vi "Intake Loop.vi"(8 "error in (no error)":errorcluster) -> ()   [LabVIEW 2014]
uses:
  Intake Control.ctl
  <vilib>/Rock Robotics/WPI/MotorControl/WPI_MotorControlDeviceRef.ctl
  <vilib>/Rock Robotics/SystemInterfaces/Typedef/FPGA_TypedefDigitalModule.ctl
  <vilib>/Rock Robotics/SystemInterfaces/DIO/FPGA_DIOPWMChannel.ctl
  <vilib>/Rock Robotics/WPI/PWM/WPI_PWMDeadband.ctl
  <vilib>/Rock Robotics/WPI/CAN/Jaguar/SubVIs/WPI_CANJaguar_ControlMode.ctl
  <vilib>/Rock Robotics/WPI/PWM/WPI_PWMTransform_ConPane.ctl
  <vilib>/Rock Robotics/WPI/Solenoid/WPI_SolenoidDevRef.ctl
  <vilib>/Rock Robotics/SystemInterfaces/Typedef/FPGA_TypedefSolenoidModule.ctl
  <vilib>/Rock Robotics/WPI/Solenoid/WPI_SolenoidChannel.ctl
  <vilib>/Rock Robotics/WPI/Solenoid/WPI_SolenoidValue.ctl
  <vilib>/Rock Robotics/Network Tables/SD Write Number.vi
  <vilib>/Rock Robotics/WPI/Solenoid/WPI_SolenoidSetEnum.vi
  <vilib>/Rock Robotics/WPI/MotorControl/WPI_MotorControlSafetyCheck.vi
  <vilib>/Rock Robotics/WPI/Solenoid/WPI_SolenoidSafetyCheck.vi
panel:
  in  "Motor Speed":dbl=1.0
  in  "Invert?":bool=TRUE
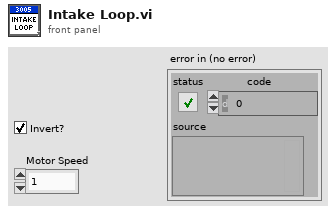
[diagram p1: front panel]
types:
  T1 = typedef "WPI_MotorControlDeviceRef.ctl" = cluster{"DeviceStatus":errorcluster, "Type":enum16{"PWM", "CAN"}, "PWM":cluster{"Digital Module":T2, "PWM Channel":T3, "DeadBand":T4}, "CAN":cluster{"Device Number":u8, "Control Mode":T5, "Semaphore":T6, "Max Vout":dbl}, "Invert":bool, "TransformRef":T7, "InvTransformRef":T7}
  T2 = typedef "FPGA_TypedefDigitalModule.ctl" = enum16{"Digital Module 1", "Digital Module 2"}
  T3 = typedef "FPGA_DIOPWMChannel.ctl" = enum8{"PWM 1", "PWM 2", "PWM 3", "PWM 4", "PWM 5", "PWM 6", "PWM 7", "PWM 8", "PWM 9", "PWM 10", "Invalid"}
  T4 = typedef "WPI_PWMDeadband.ctl" = cluster{"Name":string, "maxPositivePwm":i32, "minPositivePwm":i32, "centerPwm":i32, "maxNegativePwm":i32, "minNegativePwm":i32, "angularRange":u16}
  T5 = typedef "WPI_CANJaguar_ControlMode.ctl" = enum8{"Percent VBus", "Current", "Speed", "Position", "Voltage"}
  T6 = typedef "Semaphore RefNum" = refnum<k1>
  T7 = typedef "WPI_PWMTransform_ConPane.ctl" = refnum<vi>
  T8 = typedef "WPI_SolenoidDevRef.ctl" = cluster{"DevStatus":errorcluster, "Solenoid Module":T9, "Forward Solenoid Channel":T10, "Reverse Solenoid Channel":T10}
  T9 = typedef "FPGA_TypedefSolenoidModule.ctl" = enum16{"Solenoid Module 1", "Solenoid Module 2"}
  T10 = typedef "WPI_SolenoidChannel.ctl" = enum8{"Solenoid 1", "Solenoid 2", "Solenoid 3", "Solenoid 4", "Solenoid 5", "Solenoid 6", "Solenoid 7", "Solenoid 8", "Invalid"}
  T11 = cluster{"Intake Motor":T1, "Intake":T8, "Motor Speed":dbl, "Motor Direction":i32, "Pateadora":T8}
  T12 = typedef "Intake Control.ctl" = enum16{"Idle", "Contain", "Extend", "Motor Still", "Motor Outward", "Motor Inward", "Patea Extend", "Patea Retract"}
  T13 = typedef "WPI_SolenoidValue.ctl" = enum16{"Off", "On", "Forward", "Reverse"}
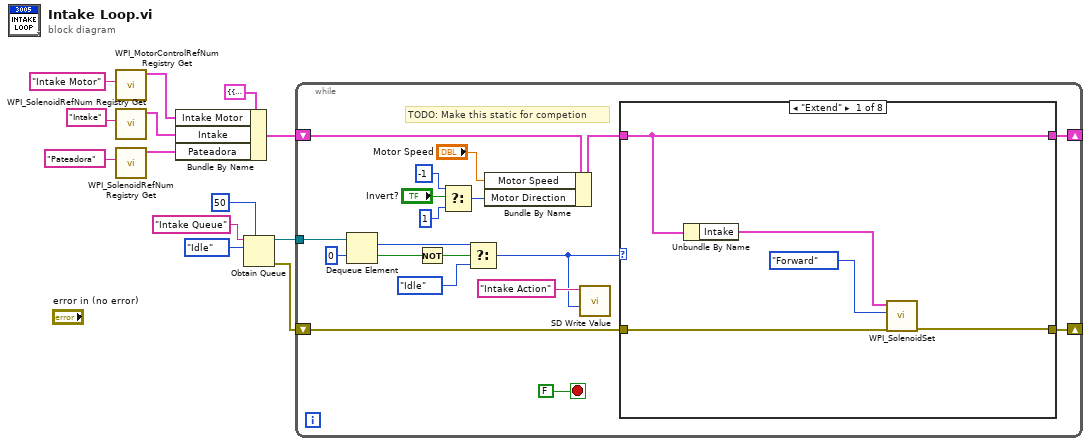
[diagram p0: block diagram]
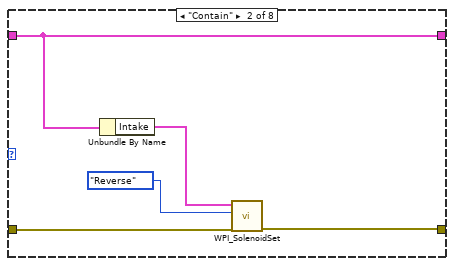
[diagram p2: hidden frame]
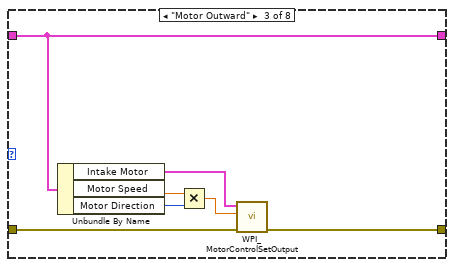
[diagram p3: hidden frame]
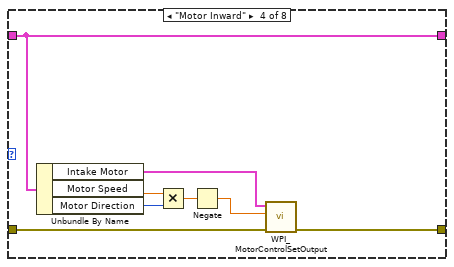
[diagram p4: hidden frame]
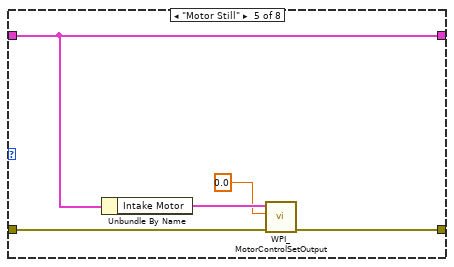
[diagram p5: hidden frame]
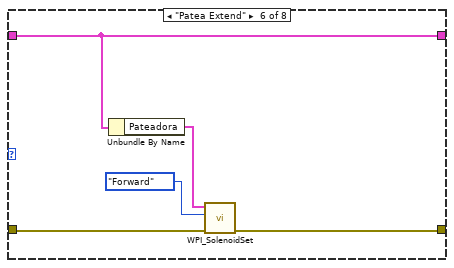
[diagram p6: hidden frame]
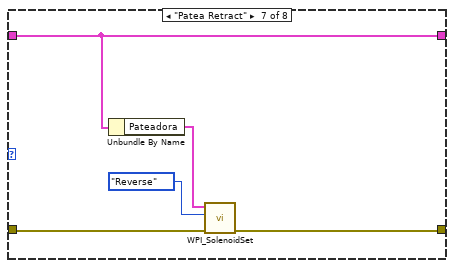
[diagram p7: hidden frame]
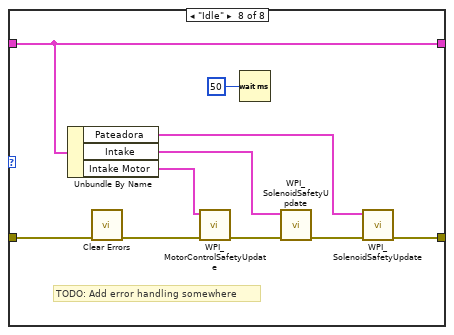
[diagram p8: hidden frame]
diagram:
  n1 = call <vilib>:"WPI_MotorControlRefNum Registry Get.vi"("refnum name"="Intake Motor") -> ("MotorControlDevRef"=w3:T1)  [unwired: 9 in, 1 out]
  n2 = call <vilib>:"WPI_SolenoidRefNum Registry Get.vi"("refnum name"="Intake") -> ("SolenoidDevRef"=w2:T8)  [unwired: 9 in, 1 out]
  n3 = call <vilib>:"WPI_SolenoidRefNum Registry Get.vi"("refnum name"="Pateadora") -> ("SolenoidDevRef"=w1:T8)  [unwired: 9 in, 1 out]
  n4 = Bundle By Name(cluster=T11 {"Intake Motor"={"DeviceStatus"={"status"=FALSE, "code"=0, "source"=""}, "Type"=enum."PWM", "PWM"={"Digital Module"=enum."Digital Module 1", "PWM Channel"=enum."Invalid", "DeadBand"={"Name"="", "maxPositivePwm"=0, "minPositivePwm"=0, "centerPwm"=0, "maxNegativePwm"=0, "minNegativePwm"=0, "angularRange"=0}}, "CAN"={"Device Number"=0, "Control Mode"=enum."Percent VBus", "Semaphore"=refnum, "Max Vout"=12.0}, "Invert"=FALSE, "TransformRef"=refnum, "InvTransformRef"=refnum}, "Intake"={"DevStatus"={"status"=FALSE, "code"=0, "source"=""}, "Solenoid Module"=enum."Solenoid Module 1", "Forward Solenoid Channel"=enum."Invalid", "Reverse Solenoid Channel"=enum."Invalid"}, "Motor Speed"=0.0, "Motor Direction"=0, "Pateadora"={"DevStatus"={"status"=FALSE, "code"=0, "source"=""}, "Solenoid Module"=enum."Solenoid Module 1", "Forward Solenoid Channel"=enum."Invalid", "Reverse Solenoid Channel"=enum."Invalid"}}, "Intake Motor"=w3, "Intake"=w2, "Pateadora"=w1) -> (w11:T11)
  n5 = Obtain Queue(max queue size (-1, unlimited)=50, name (unnamed)="Intake Queue", element data type=Intake_Control."Idle") -> (queue out=w7:refnum<queue>, error out=w10:errorcluster)  [unwired: 2 in, 1 out]
  n6 = while {
    tunnel: w7 -> [w31]
    shift-right: [w16] -> _
    shift-left: w10 -> [w22]
    shift-right: [w23] -> _
    shift-left: w11 -> [w30]
    stop <- FALSE stop-if-true
    # "TODO: Make this static for competion"
    n7 = Dequeue Element(queue=w31, timeout in ms (-1)=0) -> (element=w19:T12, timed out?=w21:bool)  [unwired: 1 in, 2 out]
    n8 = Not(x=w21) -> (.not. x?=w20:bool)
    n9 = Select(t=-1, s="Invert?", f=1) -> (s? t:f=w25:i32)
    n10 = Select(t=w19, s=w20, f=Intake_Control."Idle") -> (s? t:f=w14:T12)
    n11 = Bundle By Name(cluster=w30, "Motor Speed"="Motor Speed", "Motor Direction"=w25) -> (w29:T11)
    n12 = call-poly <vilib>:"SD Write Value.vi"("Numeric"=w14, "Name"="Intake Action" ("Table Prefix")) -> ()  [unwired: 8 in, 2 out]
    n13 = case shown="\"Extend\"" w14 {
      tunnel: [w35 w39 w48 w56 w61 w64 w69 w80] -> w16
      tunnel: w22 -> [w36 w40 w49 w57 w62 w66 w71 w82]
      tunnel: w29 -> [w37 w42 w47 w55 w60 w67 w72 w81]
      tunnel: [w37 w42 w47 w55 w60 w67 w72 w81] -> w23
      frame "Extend" {
        n14 = Unbundle By Name(w37) -> ("Intake"=w34:T8)
        n15 = call-poly <vilib>:"WPI_SolenoidSet.vi"("error in (no error)"=w36, "Value"=WPI_SolenoidValue."Forward", "SolenoidDevRef"=w34) -> ("error out"=w35:errorcluster)  [unwired: 7 in, 1 out]
      }
      frame "Contain" {
        n16 = Unbundle By Name(w42) -> ("Intake"=w41:T8)
        n17 = call-poly <vilib>:"WPI_SolenoidSet.vi"("error in (no error)"=w40, "Value"=WPI_SolenoidValue."Reverse", "SolenoidDevRef"=w41) -> ("error out"=w39:errorcluster)  [unwired: 7 in, 1 out]
      }
      frame "Motor Outward" {
        n18 = Unbundle By Name(w47) -> ("Intake Motor"=w43:T1, "Motor Speed"=w46:dbl, "Motor Direction"=w45:i32)
        n19 = Multiply(x=w46, y=w45) -> (x*y=w44:dbl)
        n20 = call <vilib>:"WPI_MotorControlSetOutput.vi"("error in (no error)"=w49, "Output"=w44, "MotorControlDevRef"=w43) -> ("error out"=w48:errorcluster)  [unwired: 6 in, 2 out]
      }
      frame "Motor Inward" {
        n21 = Unbundle By Name(w55) -> ("Intake Motor"=w52:T1, "Motor Speed"=w54:dbl, "Motor Direction"=w53:i32)
        n22 = Multiply(x=w54, y=w53) -> (x*y=w51:dbl)
        n23 = Negate(x=w51) -> (-x=w50:dbl)
        n24 = call <vilib>:"WPI_MotorControlSetOutput.vi"("error in (no error)"=w57, "Output"=w50, "MotorControlDevRef"=w52) -> ("error out"=w56:errorcluster)  [unwired: 6 in, 2 out]
      }
      frame "Motor Still" {
        n25 = Unbundle By Name(w60) -> ("Intake Motor"=w59:T1)
        n26 = call <vilib>:"WPI_MotorControlSetOutput.vi"("error in (no error)"=w62, "Output"=0.0, "MotorControlDevRef"=w59) -> ("error out"=w61:errorcluster)  [unwired: 6 in, 2 out]
      }
      frame "Patea Extend" {
        n27 = Unbundle By Name(w67) -> ("Pateadora"=w63:T8)
        n28 = call-poly <vilib>:"WPI_SolenoidSet.vi"("error in (no error)"=w66, "Value"=WPI_SolenoidValue."Forward", "SolenoidDevRef"=w63) -> ("error out"=w64:errorcluster)  [unwired: 7 in, 1 out]
      }
      frame "Patea Retract" {
        n29 = Unbundle By Name(w72) -> ("Pateadora"=w68:T8)
        n30 = call-poly <vilib>:"WPI_SolenoidSet.vi"("error in (no error)"=w71, "Value"=WPI_SolenoidValue."Reverse", "SolenoidDevRef"=w68) -> ("error out"=w69:errorcluster)  [unwired: 7 in, 1 out]
      }
      frame "Idle" {
        # "TODO: Add error handling somewhere"
        n31 = Unbundle By Name(w81) -> ("Pateadora"=w75:T8, "Intake"=w76:T8, "Intake Motor"=w77:T1)
        n32 = call <vilib>:"Clear Errors.vi"("error in (no error)"=w82) -> ("error out"=w74:errorcluster)  [unwired: 5 in, 1 out]
        n33 = call <vilib>:"WPI_MotorControlSafetyUpdate.vi"("error in (no error)"=w74, "MotorControlDevRef"=w77) -> ("error out"=w79:errorcluster)  [unwired: 9 out]
        n34 = Wait (ms)(milliseconds to wait=u32 50 ("millisecond multiple")) -> ()  [unwired: 1 out]
        n35 = call <vilib>:"WPI_SolenoidSafetyUpdate.vi"("error in (no error)"=w79, "SolenoidDevRef"=w76) -> ("error out"=w78:errorcluster)  [unwired: 9 out]
        n36 = call <vilib>:"WPI_SolenoidSafetyUpdate.vi"("error in (no error)"=w78, "SolenoidDevRef"=w75) -> ("error out"=w80:errorcluster)  [unwired: 9 out]
      }
    }
  }
